vi "通讯包应答包.vi"(9 "数据字段":string, 10 "GO/OVER":string, 11 "QN":string) -> (3 "通讯包字符串":string)   [LabVIEW 2016]
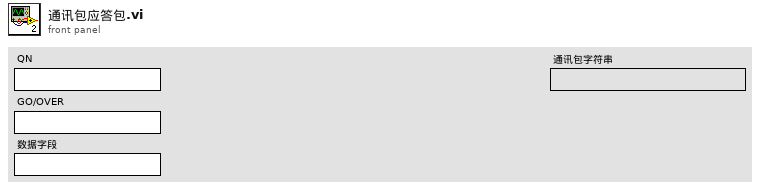
[diagram p1: front panel]
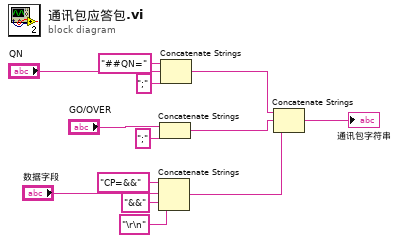
[diagram p0: block diagram]
diagram:
  n1 = Concatenate Strings("CP=&&" ("字符串"), "数据字段", "&&" ("字符串"), "\r\n" ("字符串")) -> (w2:string)
  n2 = Concatenate Strings("GO/OVER", ";" ("字符串")) -> (w3:string)
  n3 = Concatenate Strings("##QN=" ("字符串"), "QN", ";" ("字符串")) -> (w4:string)
  n4 = Concatenate Strings(w4, w3, w2) -> (→"通讯包字符串":string)
